vi "DataLog Explain Log Access Error.vi"(0 "tag log directory":path, 11 "error in":errorcluster) -> (4 "dup tag log directory":path, 15 "error out":errorcluster)   [LabVIEW 2012]
doc: "Helps explain errors that occur when performing file access on the tag log. This VI prepends a generic explanation that includes the tag log directory when a set input error is wired."
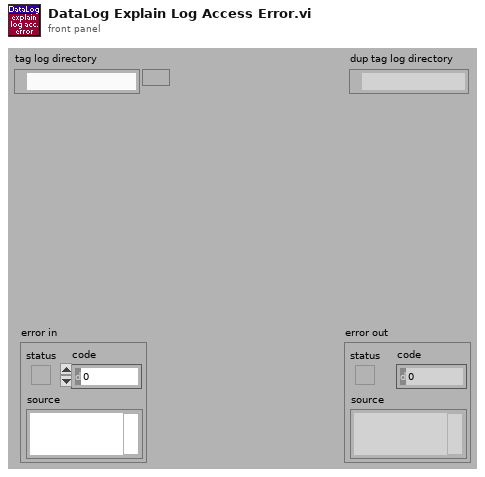
[diagram p1: front panel]
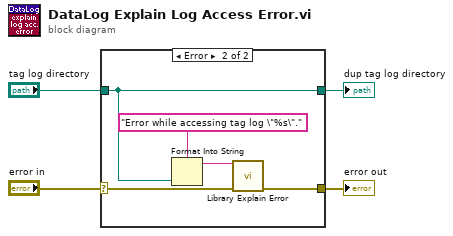
[diagram p0: block diagram]
diagram:
  n1 = case shown="Error" "error in" {
    selector: "error in" -> [w6 w11]
    tunnel: [w6 w10] -> w3
    tunnel: "tag log directory" -> [w5 w7]
    tunnel: [w5 w7] -> w1
    frame No Error {
    }
    frame Error {
      n2 = Format Into String(format string="Error while accessing tag log \"%s\".", w7) -> (resulting string=w9:string)  [unwired: 2 in, 1 out]
      n3 = call "Library Explain Error.vi"("explanation prefix (none)"=w9, "error in (no error)"=w11) -> ("explained error"=w10:errorcluster)  [unwired: 13 in]
    }
  }
  "error out" <- w3
  "dup tag log directory" <- w1
